vi "Speaker-PlaySequence.vi"(7 "Device reference":refnum<vi>, 8 "error in (no error)":errorcluster, 9 "Eventstring":string="auto-generate", 11 "Sine sequence":T1) -> (0 "error out":errorcluster)   [LabVIEW 2015]
doc: "Plays a tone (sine wave) on the speaker.\n\nDevice reference: Which speaker?\nFrequency (Hz): Tone frequency\nDuration (ms): Tone duration\nEventstring:\n empty: no timestamp\n unwired or \"auto-generate\":\n [name].play:[freq]Hz,[duration]ms\n otherwise: timestamp w/ provided string\n\nIf you try to play more than one tone at a time, they will just get queued."
uses:
  Typedefs/Speaker.ctl
  Rack/Typedefs/OutputRequest refnum.ctl
  Rack/Typedefs/OutputRequest.ctl
  Rack/Typedefs/InputData cluster.ctl
  Rack/Methods/Port drivers/DigitalInput-DataCluster.ctl
  Typedefs/Speaker - Sine sequence.ctl
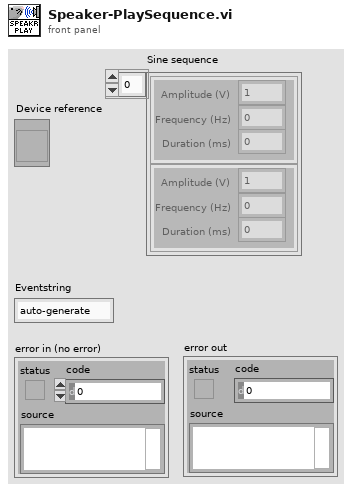
[diagram p1: front panel]
types:
  T1 = typedef "Speaker - Sine sequence.ctl" = cluster{"Frequency (Hz)":dbl, "Duration (ms)":dbl, "Amplitude (V)":dbl}[]
  T2 = typedef "Speaker.ctl" = cluster{"Settings":cluster{"Portname":string, "Index":i32, "Timestamp portname":string}, "OutputRequest event ref":T3, "InputData reference":refnum<vi>}
  T3 = typedef "OutputRequest refnum.ctl" = refnum<user-event>
  T4 = typedef "OutputRequest.ctl" = cluster{"Target":string, "Command":string}
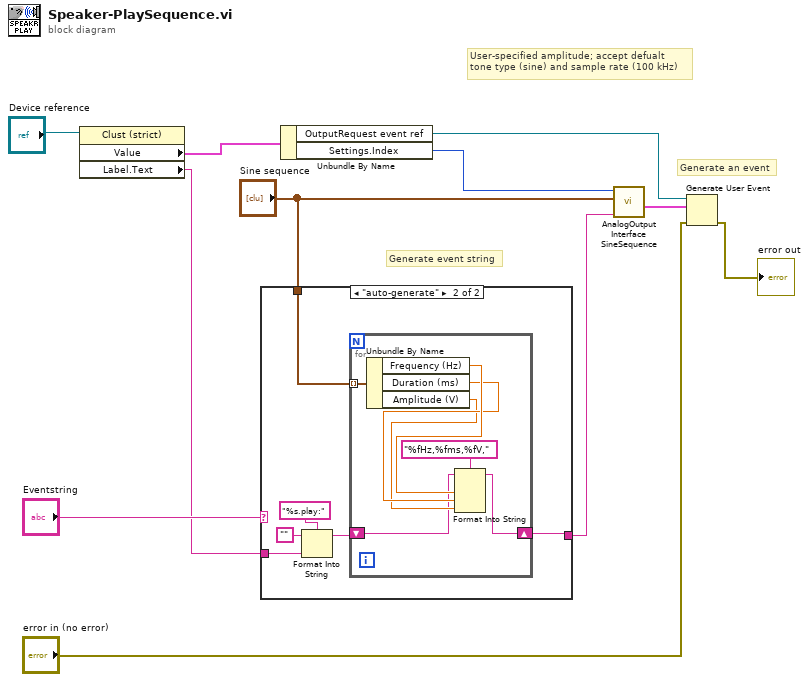
[diagram p0: block diagram]
diagram:
  # "User-specified amplitude; accept defualt\ntone type (sine) and sample rate (100 kHz)"
  # "Generate event string"
  # "Generate an event"
  n1 = property class="Clust (strict)"(reference="Device reference") -> ("Value"=w10:T2, "Label.Text"=w7:string)  [unwired: 1 in, 2 out]
  n2 = case shown="\"auto-generate\"" "Eventstring" {
    selector: "Eventstring" -> [w12 _]
    tunnel: w7 -> [_ w16]
    tunnel: [w12 w13] -> w3
    tunnel: "Sine sequence" -> [_ w15]
    frame Default {
      # "Use user-provided string"
    }
    frame "auto-generate" {
      n3 = Format Into String(format string="%s.play:", initial string="", w16) -> (resulting string=w14:string)  [unwired: 1 in, 1 out]
      n4 = for {
        tunnel: w15 -> [w24] mode=indexing
        shift-right: [w19] -> w13
        shift-left: w14 -> [w20]
        n5 = Unbundle By Name(w24) -> ("Frequency (Hz)"=w23:dbl, "Duration (ms)"=w22:dbl, "Amplitude (V)"=w21:dbl)
        n6 = Format Into String(format string="%fHz,%fms,%fV,", initial string=w20, w23, w22, w21) -> (resulting string=w19:string)  [unwired: 1 in, 1 out]
      }
    }
  }
  n7 = Unbundle By Name(w10) -> ("OutputRequest event ref"=w9:T3, "Settings.Index"=w2:i32)
  n8 = call "AnalogOutput Interface SineSequence.vi"("Eventstring"=w3, "Sine sequence"="Sine sequence", "Port index"=w2) -> ("OutputRequest"=w4:T4)  [unwired: 8 in]
  n9 = Generate User Event(user event=w9, event data cluster=w4, error in="error in (no error)") -> (error out=→"error out":errorcluster)  [unwired: 1 in, 1 out]
